vi "Cleanup.vi"(8 "error in (no error)":errorcluster, 11 "Dual Relay Bricklet in":refnum<class "Dual Relay Bricklet.lvclass">) -> (0 "error out":errorcluster)   [LabVIEW 2011, in "Tinkerforge.lvlib" / "Dual Relay Bricklet.lvclass"]
doc: "This VI is the child implementation of \"Cleanup.vi\" and releases all synchronization objects of this child object."
uses:
  Dual Relay Bricklet.lvclass
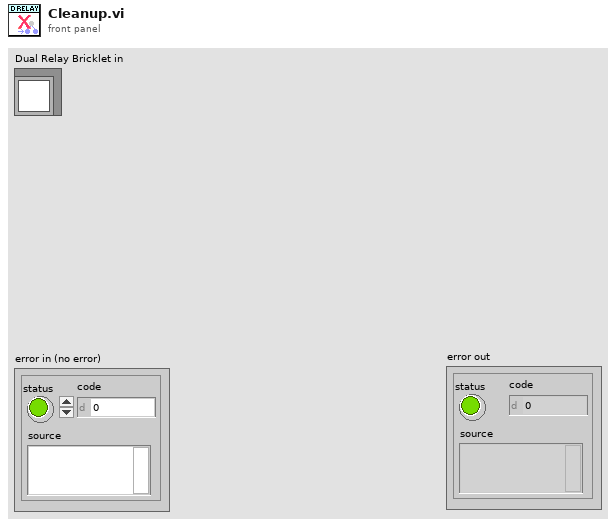
[diagram p1: front panel]
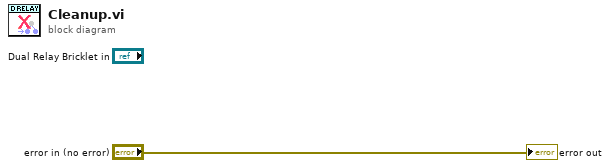
[diagram p0: block diagram]
diagram:
  "error out" <- "error in (no error)"
